vi "act_avb_shutoff.vi"   [LabVIEW 2018]
uses:
  <vilib>/rvi/DataTransferAndStorage/Container/Common/niFpgaContainerExecOnDevCompGetState.vi
  <vilib>/rvi/Emulation/niFpgaEmulationIsFPGAContextNoSignature.vi
  <vilib>/rvi/DataTransferAndStorage/Container/Common/niFpgaContainerGetUniqueNameForEmu.vi
  <vilib>/rvi/Memory/Memory_Emulation/niFpgaMemoryEmulationCacheClearOnFirstRun.vi
  <vilib>/rvi/Memory/Memory_Emulation/nirvimemoryEmulationManagerCache_MakeExclusive.vi
  <vilib>/rvi/Memory/Memory_Emulation/niFpgaMemoryEmulationValidateCache.vi
  <vilib>/rvi/Memory/Memory_Emulation/nirvimemoryEmulationManagerCache_InsertValue.vi
  <vilib>/Utility/error.llb/Clear Errors.vi
  <vilib>/rvi/Memory/Memory_Emulation/nirvimemoryEmulationManagerCache_ReleaseExclusive.vi
  <vilib>/rvi/Memory/Memory_Emulation/nirvimemoryEmulationManagerCache_GetValue.vi
  <vilib>/rvi/Memory/Memory_Emulation/nirvimemoryEmulationManagerCache_SetValue.vi
  <vilib>/rvi/Emulation/niFpgaProcessEmulError.vi
  <vilib>/rvi/Emulation/niFpgaSctlEmulationGetInTimedLoop.vi
  <vilib>/rvi/eio/common/nirviEmuTemplateMethod_errors.vi
  <vilib>/rvi/DataTransferAndStorage/Container/XNode/niFpgaContainer.xnode
  <vilib>/rvi/DataTransferAndStorage/Register/Emulation/niFpgaRegisterEmulationRefIn.vi
  <vilib>/eio/EIONode/EIONode.xnode
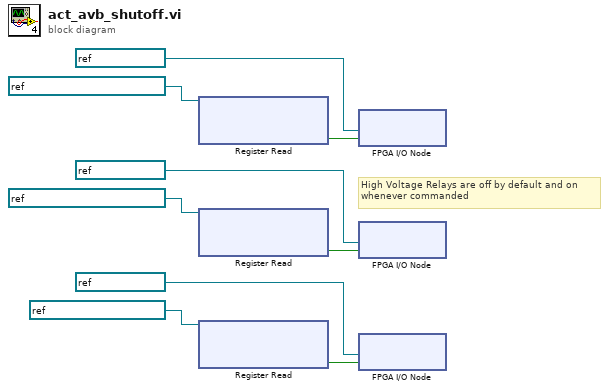
[diagram p0: block diagram]
diagram:
  # "High Voltage Relays are off by default and on\nwhenever commanded"
  n1 = xnode "Register Read"("Register In"=refnum<k21> "REG_avb_shutoff_prim_1") -> ("Data"=w7:bool)  [unwired: 1 out]
  n2 = xnode "Register Read"("Register In"=refnum<k21> "REG_avb_shutoff_prim_2") -> ("Data"=w4:bool)  [unwired: 1 out]
  n3 = xnode "Register Read"("Register In"=refnum<k21> "REG_avb_shutoff_res") -> ("Data"=w1:bool)  [unwired: 1 out]
  n4 = xnode "FPGA I/O Node"("I/O Item"=w7, "FPGA I/O In"=refnum<k21> "Mod2/DIO6") -> ()  [unwired: 1 out]
  n5 = xnode "FPGA I/O Node"("I/O Item"=w4, "FPGA I/O In"=refnum<k21> "Mod2/DIO7") -> ()  [unwired: 1 out]
  n6 = xnode "FPGA I/O Node"("I/O Item"=w1, "FPGA I/O In"=refnum<k21> "Mod2/DIO8") -> ()  [unwired: 1 out]
